vi "test harness_FXP_Linear_controller_observer.vi"(8 "error in (no error)":errorcluster, 11 "TestCase in":refnum<class "FXP_observer_TestCase.lvclass">) -> (0 "error out":errorcluster, 3 "TestCase out":refnum<class "FXP_observer_TestCase.lvclass">)   [LabVIEW 2017, in "FXP_observer_TestCase.lvclass"]
uses:
  FXP_observer_TestCase.lvclass
  C:/Program Files (x86)/National Instruments/LabVIEW 2017/vi.lib/addons/_JKI Toolkits/VI Tester/TestCase.llb/TestCase.lvclass
  fpga_VIs/fpga_subVIs_ssxy/fixed-point-ss/typeDefs/FXPControlParams_distEst.ctl
  fpga_VIs/fpga_subVIs_ssxy/fixed-point-ss/typeDefs/x_vec_type.ctl
  <vilib>/rvi/DesktopExecutionNode/Execution/niFpgaDEN_Execute.vi
  <vilib>/rvi/DesktopExecutionNode/DesktopExecutionNode.xnode
  <userlib>/_VITAC/VITAC.lvlib
panel:
  out "A_mat":dbl[][](array[numeric])
  out "A*xk(out)":fxp<+/-,32,5>[](array[numeric])
  out "A*x(expected)":T1
  out "xk_1_0":T1
  out "uk (expected)":fxp<+/-,64,12>
  out "deltaUk (expected)":fxp<+/-,64,12>
  in  "d_hat":fxp<+/-,32,6>
  out "Ns_obs/cntrl":u8
  in  "ControlParams_distEst":T2={"umax"=3.0, "Ns_obs/cntrl"=22, "ref_f_VEC"=[0.0, 0.0], "du_max"=5.0, "Nbar"=0.0}
  out "error A*x_k_1":errorcluster
  out "del u(k)":fxp<+/-,64,15>
  out "u_k (saturated)":fxp<+/-,32,5>
  out "error (xk_0_1)":errorcluster
  out "error (ydest)":errorcluster
  in  "x_u(k)":fxp<+/-,32,8>
  in  "y(k)":fxp<+/-,18,5>=0.123046875
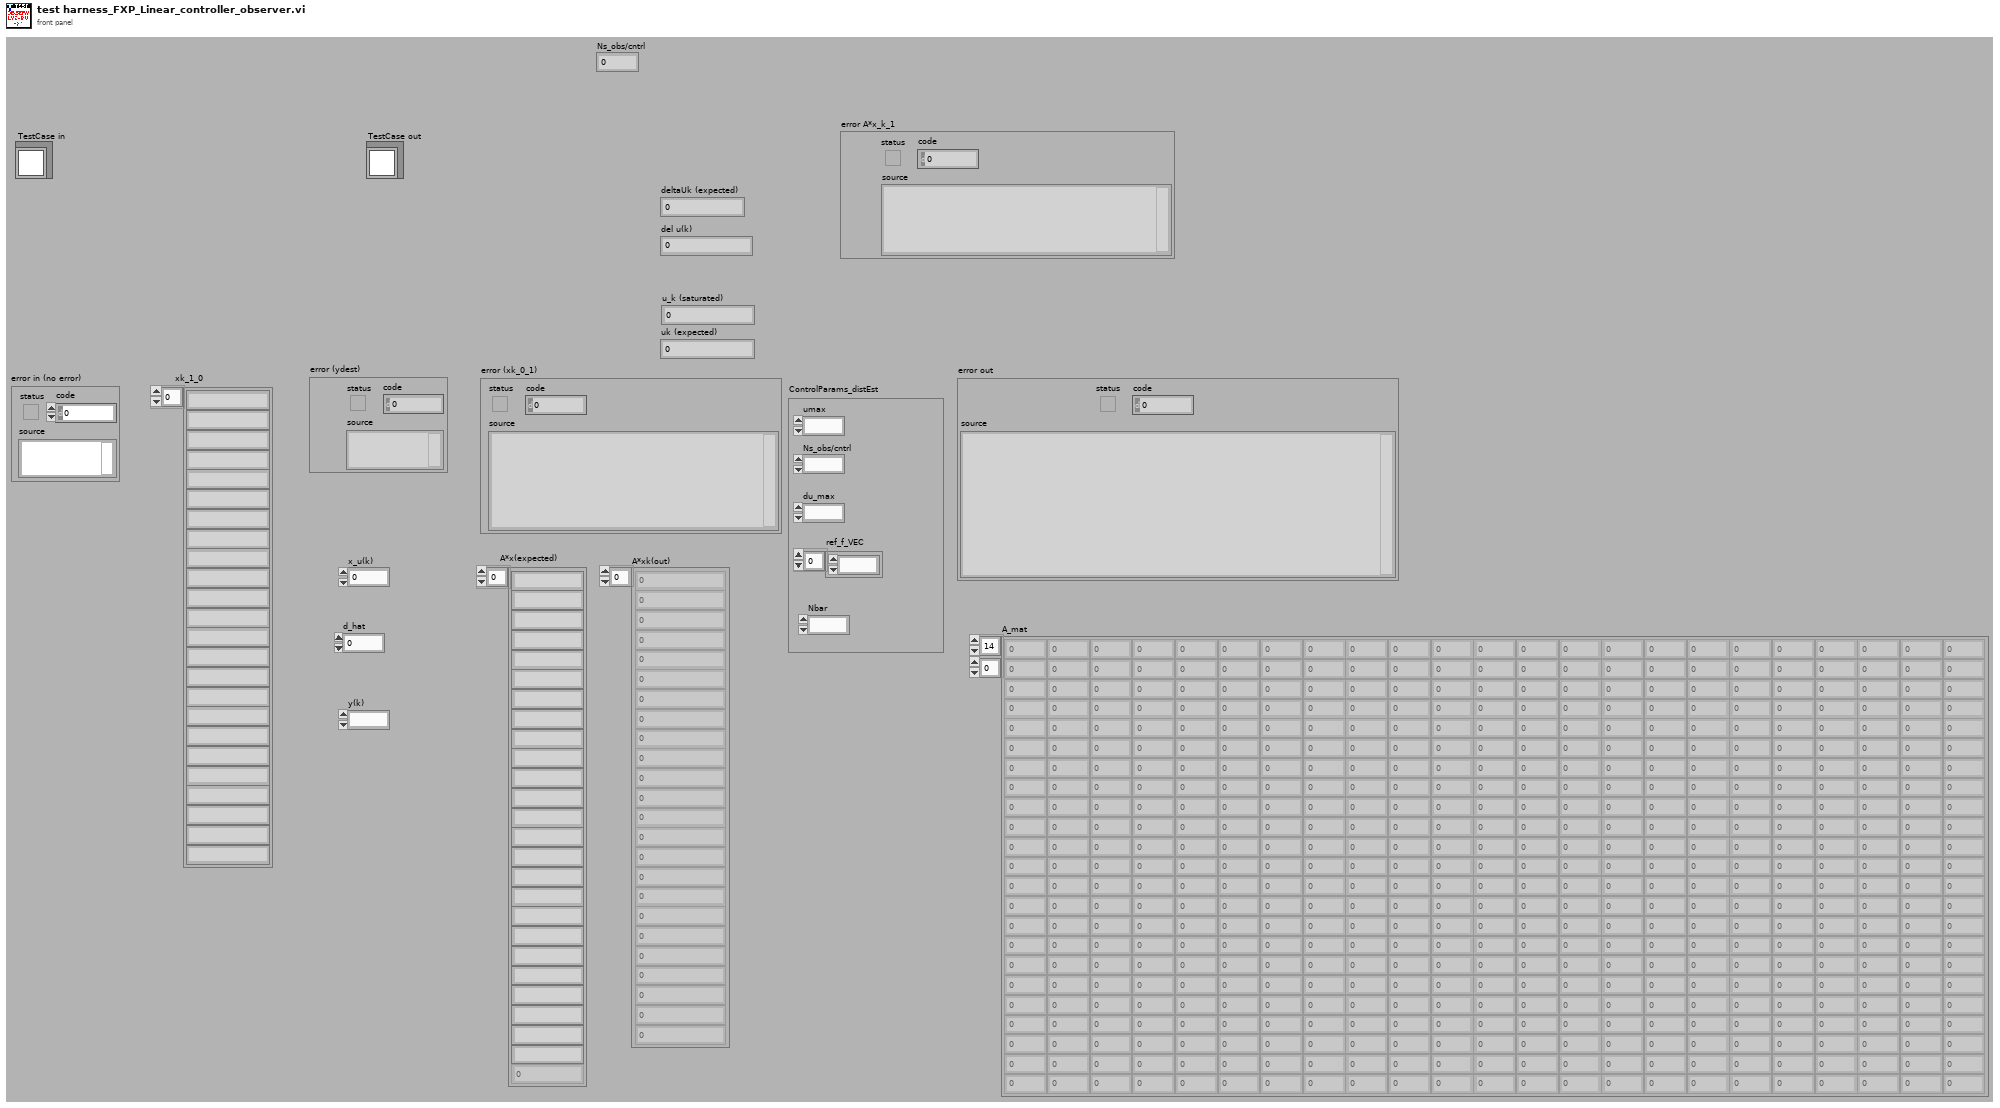
[diagram p1: front panel]
types:
  T1 = typedef "x_vec_type.ctl" = fxp<+/-,32,6>[]
  T2 = typedef "FXPControlParams_distEst.ctl" = cluster{"umax":fxp<+/-,18,5>, "Ns_obs/cntrl":u8, "ref_f_VEC":fxp<+/-,32,5>[], "du_max":fxp<+/-,18,5>, "Nbar":fxp<+/-,32,5>}
  T3 = typedef "UT_matrix_data.ctl" = cluster{"Bz":T4[], "Ldist":T5[], "Kz":T6[], "Nx":T7[], "Ax_col":T8[], "X_vec":T9[], "Cz":T10[]}
  T4 = typedef "Bz_vec_scalar.ctl" = fxp<+/-,32,3>
  T5 = typedef "Lz_vec_scalar.ctl" = fxp<+/-,32,3>
  T6 = typedef "Kz_vec_scalar.ctl" = fxp<+/-,32,10>
  T7 = typedef "Nx_vec_scalar.ctl" = fxp<+/-,32,2>
  T8 = typedef "Az_vec_scalar.ctl" = fxp<+/-,32,7>
  T9 = typedef "x_vec_scalar.ctl" = fxp<+/-,32,6>
  T10 = typedef "Cz_vec_scalar.ctl" = fxp<+/-,32,4>
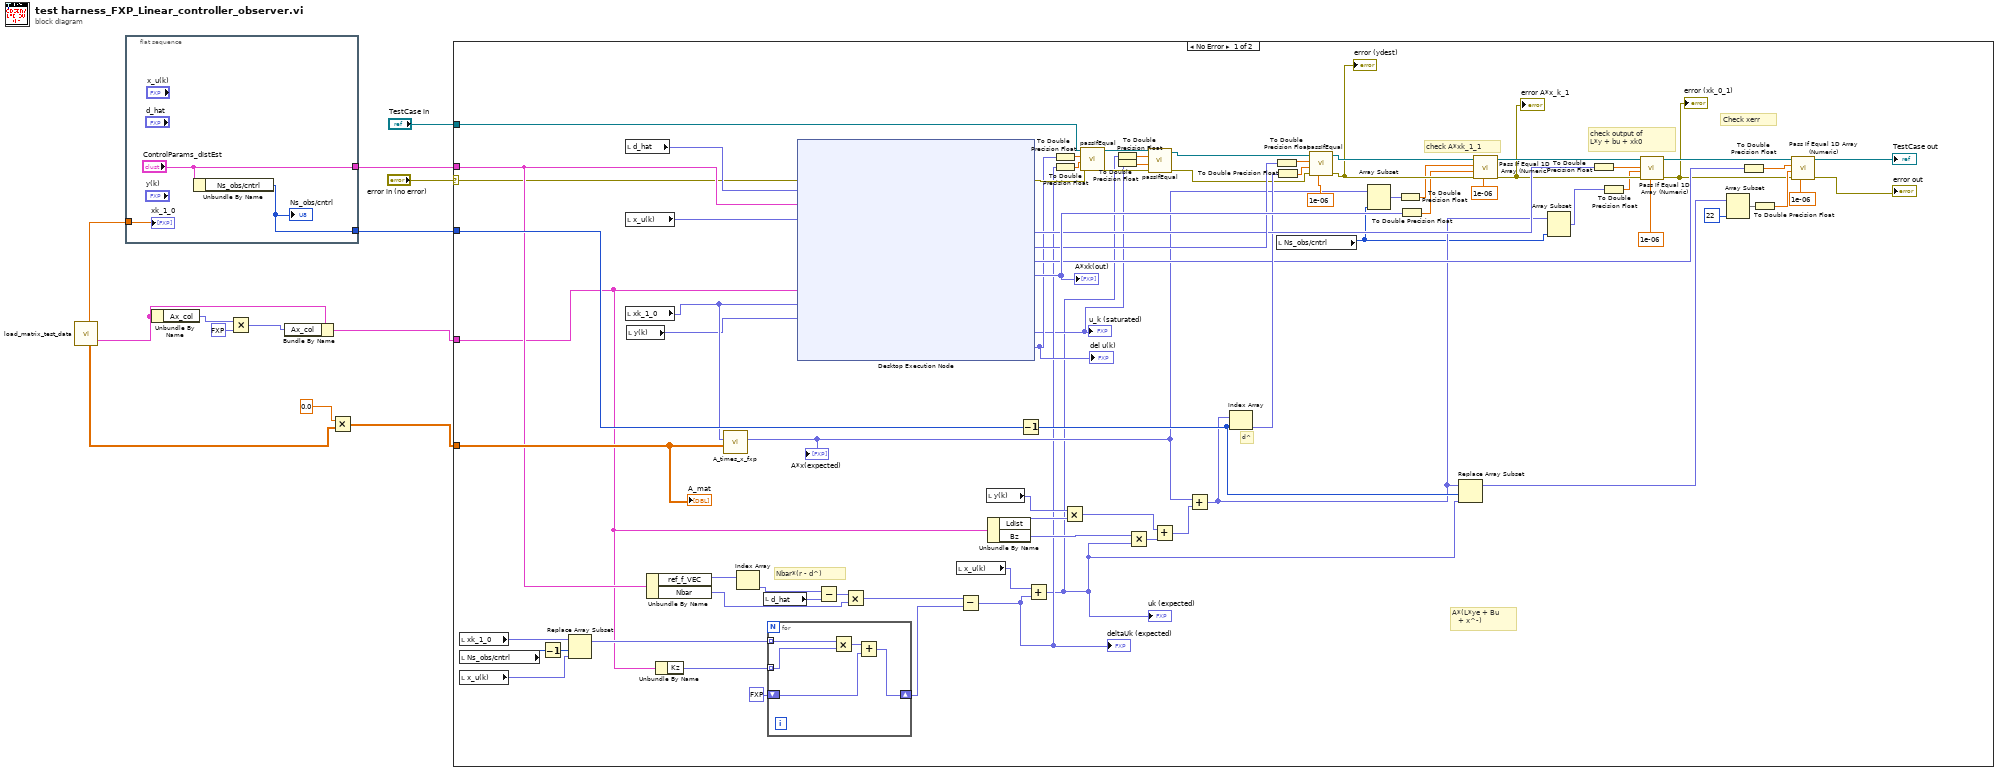
[diagram p0: block diagram]
diagram:
  n1 = call "load_matrix_test_data.vi"() -> ("A_mat"=w8:dbl[][], "X_test"=w10:dbl[], "output cluster"=w3:T3)  [unwired: 4 in, 5 out]
  n2 = flat-sequence {
    tunnel: [w16] -> w12
    tunnel: ["ControlParams_distEst"] -> w11
    tunnel: w10 -> [w14]
    frame #0 {
      n3 = Unbundle By Name("ControlParams_distEst") -> ("Ns_obs/cntrl"=w16:u8)
      "Ns_obs/cntrl" <- w16
      "xk_1_0" <- w14
    }
  }
  n4 = Unbundle By Name(w3) -> ("Ax_col"=w5:T8[])
  n5 = Multiply(x=w5, y=fxp<+,32,5> 0.0) -> (x*y=w2:fxp<+/-,64,12>[])
  n6 = Bundle By Name(cluster=w3, "Ax_col"=w2) -> (w1:T3)
  n7 = Multiply(x=0.0, y=w8) -> (x*y=w7:dbl[][])
  n8 = case shown="No Error" "error in (no error)" {
    selector: "error in (no error)" -> [w38 _]
    tunnel: w7 -> [w94 _]
    tunnel: "TestCase in" -> [w29 _]
    tunnel: w12 -> [w85 _]
    tunnel: w11 -> [w68 _]
    tunnel: w1 -> [w48 _]
    frame No Error {
      # "Nbar*(r - d^)"
      # "d^"
      # "A*(L*ye + Bu\n   + x^-)"
      # "check A*xk_1_1"
      # "check output of \nL*y + bu + xk0"
      # "Check xerr"
      n9 = local read "xk_1_0"() -> (w53:T1)
      n10 = local read "Ns_obs/cntrl"() -> (w49:u8)
      n11 = local read "x_u(k)"() -> (w52:fxp<+/-,32,8>)
      n12 = Decrement(x=w49) -> (x-1=w50:u8)
      n13 = Replace Array Subset(array=w53, new element=w52, index=w50) -> (w51:T1)
      n14 = local read "d_hat"() -> (w54:fxp<+/-,32,6>)
      n15 = local read "x_u(k)"() -> (w62:fxp<+/-,32,8>)
      n16 = local read "xk_1_0"() -> (w65:T1)
      n17 = local read "y(k)"() -> (w46:fxp<+/-,18,5>)
      n18 = Unbundle By Name(w68) -> ("ref_f_VEC"=w74:fxp<+/-,32,5>[], "Nbar"=w67:fxp<+/-,32,5>)
      n19 = Unbundle By Name(w48) -> ("Kz"=w87:T6[])
      n20 = call "A_times_x_fxp.vi"("Az_mat in"=w94, "x_vec"=w65) -> ("A*x"=w41:T1)  [unwired: 8 in, 1 out]
      "A*x(expected)" <- w41
      n21 = Index Array(array=w74) -> (element=w73:fxp<+/-,32,5>)  [unwired: 1 in]
      n22 = local read "d_hat"() -> (w66:fxp<+/-,32,6>)
      n23 = for {
        tunnel: w51 -> [w95] mode=indexing
        tunnel: w87 -> [w99] mode=indexing
        shift-right: [w96] -> w63
        shift-left: fxp<+,32,5> 0.0 -> [w97]
        n24 = Multiply(x=w95, y=w99) -> (x*y=w98:fxp<+/-,64,16>)
        n25 = Add(x=w98, y=w97) -> (x+y=w96:fxp<+/-,32,16>)
      }
      n26 = xnode "Desktop Execution Node"("Error In"=w38, "d_hat"=w54, "ControlParams_distEst"=w68, "x_u(k)"=w62, "matrix_data"=w48, "xk_1_0"=w65, "y(k-1)"=w46) -> ("Error Out"=w30:errorcluster, "xk_0_1"=w72:fxp<+/-,32,5>[], "yd_est"=w90:fxp<+/-,32,5>, "xk_0_2"=w42:fxp<+/-,32,5>[], "A*xk(out)"=w93:fxp<+/-,32,5>[], "u_k (saturated)"=w18:fxp<+/-,32,5>, "del u(k)"=w26:fxp<+/-,64,15>)
      "u_k (saturated)" <- w18
      "del u(k)" <- w26
      "A*xk(out)" <- w93
      n27 = Subtract(x=w73, y=w66) -> (x-y=w88:fxp<+/-,34,7>)
      n28 = Multiply(x=w88, y=w67) -> (x*y=w64:fxp<+/-,64,11>)
      n29 = local read "x_u(k)"() -> (w61:fxp<+/-,32,8>)
      n30 = Subtract(x=w64, y=w63) -> (x-y=w25:fxp<+/-,32,5>)
      "deltaUk (expected)" <- w25
      n31 = local read "y(k)"() -> (w47:fxp<+/-,18,5>)
      n32 = Unbundle By Name(w48) -> ("Ldist"=w59:T5[], "Bz"=w60:T4[])
      n33 = Decrement(x=w85) -> (x-1=w45:u8)
      n34 = Add(x=w61, y=w25) -> (x+y=w17:fxp<+/-,32,5>)
      "uk (expected)" <- w17
      n35 = To Double Precision Float(number=w26) -> (double precision float=w28:dbl)
      n36 = To Double Precision Float(number=w25) -> (double precision float=w27:dbl)
      n37 = Multiply(x=w47, y=w59) -> (x*y=w57:fxp<+/-,64,10>[])
      n38 = call-dynamic "passIfEqual.vi"("error in (no error)"=w30, "y"=w27, "x"=w28, "TestCase in"=w29) -> ("error out"=w21:errorcluster, "TestCase out"=w24:refnum<class "FXP_observer_TestCase.lvclass">)  [unwired: 6 in]
      n39 = To Double Precision Float(number=w17) -> (double precision float=w20:dbl)
      n40 = To Double Precision Float(number=w18) -> (double precision float=w19:dbl)
      n41 = Multiply(x=w60, y=w17) -> (x*y=w58:fxp<+/-,64,10>[])
      n42 = call-dynamic "passIfEqual.vi"("error in (no error)"=w21, "y"=w19, "x"=w20, "TestCase in"=w24) -> ("error out"=w22:errorcluster, "TestCase out"=w23:refnum<class "FXP_observer_TestCase.lvclass">)  [unwired: 6 in]
      n43 = Add(x=w57, y=w58) -> (x+y=w56:fxp<+/-,32,8>[])
      n44 = Add(x=w41, y=w56) -> (x+y=w39:T1)
      n45 = Index Array(array=w39, index=w45) -> (element=w55:fxp<+/-,32,6>)
      n46 = To Double Precision Float(number=w90) -> (double precision float=w92:dbl)
      n47 = To Double Precision Float(number=w55) -> (double precision float=w91:dbl)
      n48 = local read "Ns_obs/cntrl"() -> (w31:u8)
      n49 = call-dynamic "passIfEqual.vi"("delta (optional)"=1e-06 ("del u_x"), "error in (no error)"=w22, "y"=w91, "x"=w92, "TestCase in"=w23) -> ("error out"=w83:errorcluster, "TestCase out"=w84:refnum<class "FXP_observer_TestCase.lvclass">)  [unwired: 5 in]
      "error (ydest)" <- w83
      n50 = Array Subset(array=w41, length=w31) -> (w71:fxp<+/-,32,6>[])  [unwired: 1 in]
      n51 = To Double Precision Float(number=w71) -> (double precision float=w32:dbl[])
      n52 = To Double Precision Float(number=w93) -> (double precision float=w33:dbl[])
      n53 = Replace Array Subset(array=w39, new element=w17, index=w45) -> (w44:T1)
      n54 = call <userlib>:"Pass If Equal 1D Array (Numeric).vi"("delta (optional)"=1e-06 ("del u_x"), "error in (no error)"=w83, "actual"=w33, "expected"=w32, "TestCase in"=w84) -> ("error out"=w36:errorcluster, "TestCase out"=w81:refnum<class "FXP_observer_TestCase.lvclass">)  [unwired: 5 in]
      "error A*x_k_1" <- w36
      n55 = Array Subset(array=w39, length=w31) -> (w40:fxp<+/-,32,6>[])  [unwired: 1 in]
      n56 = To Double Precision Float(number=w72) -> (double precision float=w34:dbl[])
      n57 = To Double Precision Float(number=w40) -> (double precision float=w35:dbl[])
      n58 = call <userlib>:"Pass If Equal 1D Array (Numeric).vi"("delta (optional)"=1e-06 ("del u_x"), "error in (no error)"=w36, "actual"=w35, "expected"=w34, "TestCase in"=w81) -> ("error out"=w37:errorcluster, "TestCase out"=w78:refnum<class "FXP_observer_TestCase.lvclass">)  [unwired: 5 in]
      "error (xk_0_1)" <- w37
      n59 = Array Subset(array=w44, length=22) -> (w70:fxp<+/-,32,6>[])  [unwired: 1 in]
      n60 = To Double Precision Float(number=w42) -> (double precision float=w43:dbl[])
      n61 = To Double Precision Float(number=w70) -> (double precision float=w76:dbl[])
      n62 = call <userlib>:"Pass If Equal 1D Array (Numeric).vi"("delta (optional)"=1e-06 ("del u_x"), "error in (no error)"=w37, "actual"=w76, "expected"=w43, "TestCase in"=w78) -> ("error out"=→"error out":errorcluster, "TestCase out"=→"TestCase out":refnum<class "FXP_observer_TestCase.lvclass">)  [unwired: 5 in]
      "A_mat" <- w94
    }
    frame Error {
    }
  }
